vi "MT Generate FSK Synchronization Parameters (number array).vi"(0 "FSK system parameters":T1={"samples per symbol (16)"=16, "symbol map"=[], "symbol phase continuity"=enum."continuous"} {"symbol map" format="%.2f"}, 5 "sync numbers":i32[](array[numeric]) format="%.0x", 7 "bits per sync number":i32=32, 11 "error in (no error)":errorcluster, 12 "expected sync location (symbols)":i32=-1, 13 "sync location uncertainty (symbols)":i32=10, 14 "sync indent (symbols)":i32) -> (4 "FSK synchronization parameters":T2 {"sync sequence" format="%.2f"}, 15 "error out":errorcluster)   [LabVIEW 2020, in "niDMT.lvlib"]
doc: "This polymorphic instance generates synchronization parameters for FSK demodulation using a synchronization sequence defined by a <B>sync numbers</B> array in which each number represents a group of bits."
uses:
  <vilib>/addons/Modulation/niDMT.lvlib
  <vilib>/addons/Modulation/niAMT.lvlib
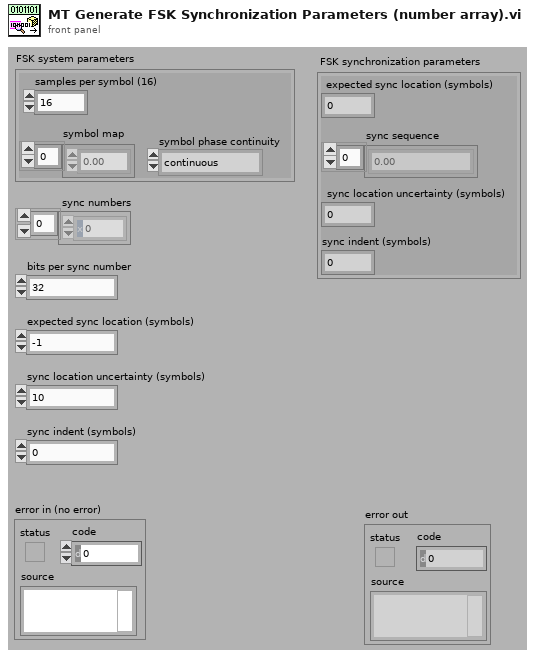
[diagram p1: front panel]
types:
  T1 = cluster{"samples per symbol (16)":i32, "symbol map":dbl[], "symbol phase continuity":enum16{"continuous", "discontinuous"}}
  T2 = cluster{"expected sync location (symbols)":i32, "sync sequence":cdb[], "sync location uncertainty (symbols)":i32, "sync indent (symbols)":i32}
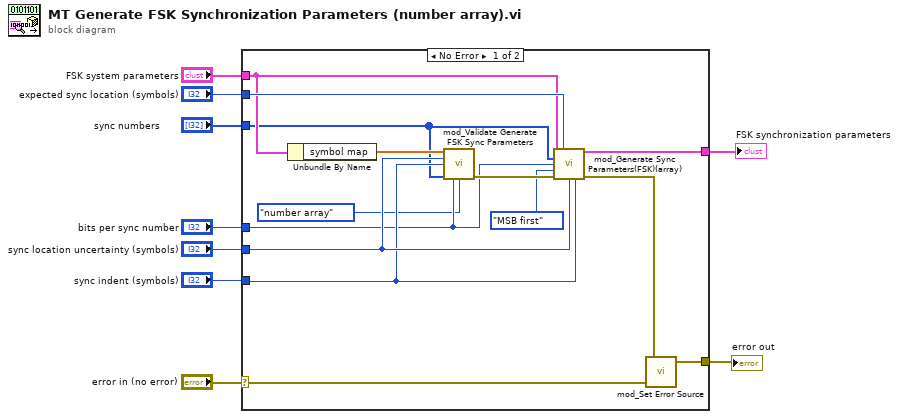
[diagram p0: block diagram]
diagram:
  n1 = case shown="No Error" "error in (no error)" {
    selector: "error in (no error)" -> [w22 w24]
    tunnel: "FSK system parameters" -> [w17 _]
    tunnel: "expected sync location (symbols)" -> [w19 _]
    tunnel: "sync location uncertainty (symbols)" -> [w15 _]
    tunnel: "sync indent (symbols)" -> [w14 _]
    tunnel: "sync numbers" -> [w13 _]
    tunnel: "bits per sync number" -> [w12 _]
    tunnel: [w23 w24] -> w2
    tunnel: [w21 _] -> w1
    frame No Error {
      n2 = Unbundle By Name(w17) -> ("symbol map"=w16:dbl[])
      n3 = call <vilib>:"mod_Validate Generate FSK Sync Parameters.vi"("symbol map"=w16, "sync location uncertainty (symbols)"=w15, "sync indent (symbols)"=w14, "sync numbers"=w13, "number of bits (or) bits per number"=w12, "sync bits specification"=enum16{"bit array", "number array", "number"}."number array") -> ("error out"=w18:errorcluster)  [unwired: 1 in, 8 out]
      n4 = call <vilib>:"mod_Generate Sync Parameters(FSK)(array).vi"("FSK system parameters"=w17, "numbers"=w13, "bits per number"=w12, "bit order"=enum16{"MSB first", "LSB first"}."MSB first", "error in (no error)"=w18, "expected sync location (symbols)"=w19, "sync location uncertainty (symbols)"=w15, "sync indent (symbols)"=w14) -> ("FSK synchronization parameters"=w21:T2, "error out"=w20:errorcluster)  [unwired: 6 out]
      n5 = call <vilib>:"mod_Set Error Source.vi"("initial error in (no error)"=w22, "final error in (no error)"=w20) -> ("error out"=w23:errorcluster)  [unwired: 3 out]
    }
    frame Error {
    }
  }
  "FSK synchronization parameters" <- w1
  "error out" <- w2
